vi "Get UI Details.vi"() -> ()   [LabVIEW 2021, in "audio_adc_frequencyResponseMeasurement.lvlib"]
uses:
  audio_adc_frequencyResponseMeasurement.lvlib
  <vilib>/MeasurementLink/MeasurementLink Measurement Server/Helpers/TypeDefs/UI Information.ctl
  <vilib>/MeasurementLink/MeasurementLink Measurement Server/MeasurementLink Measurement Server.lvlib
panel:
  out "error out":errorcluster
  in  "error in":errorcluster
  out "UI Details":T1[](array[typedef])
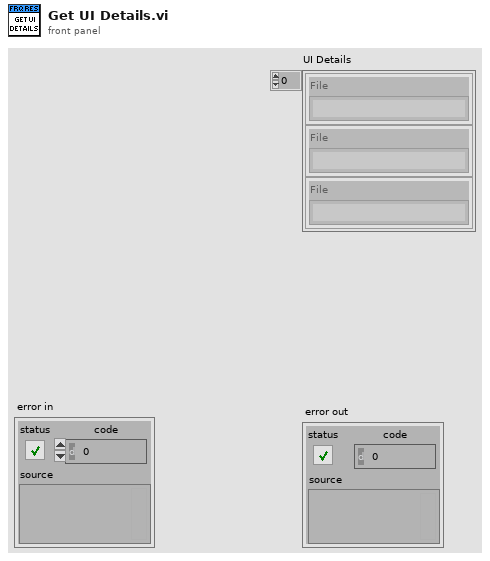
[diagram p1: front panel]
types:
  T1 = typedef "MeasurementLink Measurement Server.lvlib/UI Information.ctl" = cluster{"File":string}
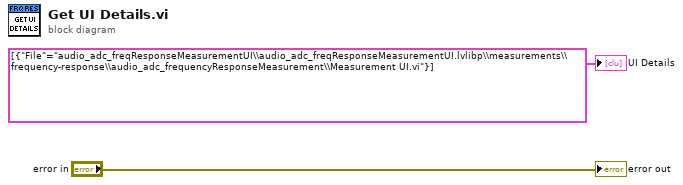
[diagram p0: block diagram]
diagram:
  "UI Details" <- T1[] [{"File"="audio_adc_freqResponseMeasurementUI\\audio_adc_freqResponseMeasurementUI.lvlibp\\measurements\\frequency-response\\audio_adc_frequencyResponseMeasurement\\Measurement UI.vi"}] ("UI Details")
  "error out" <- "error in"
